vi "Get Channel References.vi"(8 "error in (no error)":errorcluster, 10 "Dependent Node Ref":T1 format="%.0x", 11 "Section Ref in":T1 format="%.0x") -> (0 "error out":errorcluster, 2 "Array":T2[](array[typedef]) format="%.0x", 3 "Section Ref out":T1 format="%.0x")   [LabVIEW 2013, in "OPC UA Client System Explorer.lvlib"]
uses:
  OPC UA Client System Explorer.lvlib
  <vilib>/NI Veristand/Custom Device API/Custom Device Item Ref.ctl
  <vilib>/NI Veristand/Custom Device API/Data Reference.ctl
  <vilib>/NI Veristand/Custom Device API/Data Access Type.ctl
  <vilib>/NI Veristand/Custom Device API/Custom Device API.lvlib
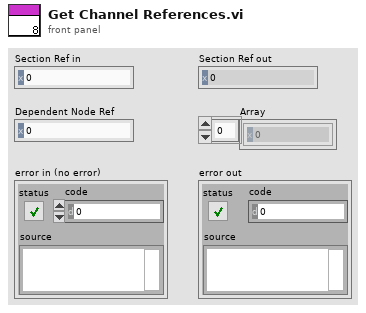
[diagram p1: front panel]
types:
  T1 = typedef "Custom Device API.lvlib/Custom Device Item Ref.ctl" = u64
  T2 = typedef "Custom Device API.lvlib/Data Reference.ctl" = i32
  T3 = typedef "Custom Device API.lvlib/Data Access Type.ctl" = enum16{"Read", "Write"}
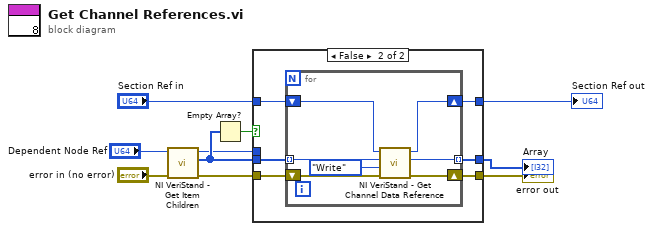
[diagram p0: block diagram]
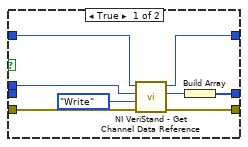
[diagram p2: hidden frame]
diagram:
  n1 = call <vilib>:"NI VeriStand - Get Item Children.vi"("error in (no error)"="error in (no error)", "Item Ref in"="Dependent Node Ref") -> ("error out"=w6:errorcluster, "Child Refs"=w10:T1[], "Item Ref out"=w8:T1)  [unwired: 6 in, 1 out]
  n2 = Empty Array?(array=w10) -> (empty?=w9:bool)
  n3 = case shown="False" w9 {
    tunnel: [w17 w24] -> w1
    tunnel: "Section Ref in" -> [w16 w23]
    tunnel: [w11 w20] -> w3
    tunnel: [w14 w22] -> w4
    tunnel: w6 -> [w13 w21]
    tunnel: w8 -> [w12 _]
    tunnel: w10 -> [_ w19]
    frame True {
      n4 = call <vilib>:"NI VeriStand - Get Channel Data Reference.vi"("error in (no error)"=w13, "Access"=Data_Access_Type."Write", "Channel Ref in"=w12, "Device Ref in"=w16) -> ("error out"=w17:errorcluster, "Channel Data Reference"=w15:T2, "Device Ref out"=w14:T1)  [unwired: 5 in]
      n5 = Build Array(w15) -> (w11:T2[])
    }
    frame False {
      n6 = for {
        tunnel: w19 -> [w26] mode=indexing
        tunnel: [w25] -> w20 mode=indexing
        shift-right: [w30] -> w24
        shift-left: w21 -> [w27]
        shift-right: [w28] -> w22
        shift-left: w23 -> [w29]
        n7 = call <vilib>:"NI VeriStand - Get Channel Data Reference.vi"("error in (no error)"=w27, "Access"=Data_Access_Type."Write", "Channel Ref in"=w26, "Device Ref in"=w29) -> ("error out"=w30:errorcluster, "Channel Data Reference"=w25:T2, "Device Ref out"=w28:T1)  [unwired: 5 in]
      }
    }
  }
  "Section Ref out" <- w4
  "Array" <- w3
  "error out" <- w1
